vi "LVClass_CameraSet GetGenericParameterBoolValue.vi"(0 "CameraSet.lvclass":refnum<class "CameraSet.lvclass">, 5 "parameter_name":string, 7 "DefaultFactorySet":bool, 11 "error in (no error)":errorcluster) -> (4 "CameraSet.lvclass":refnum<class "CameraSet.lvclass">, 6 "Value":bool, 15 "error out":errorcluster)   [LabVIEW 2020, in "CameraSet.lvclass"]
doc: "Camera parameter value getter for parameter of type boolean.\n\n<B>camera_setIn</B> : CameraSet object.\n<B>camera_setOut</B> : CameraSet object.\n<B>parameter_name</B> : Parameter name.\n<B>value</B> : Parameter value."
uses:
  CameraSet.lvclass
  CameraSet.lvclass/CameraSet.ctl
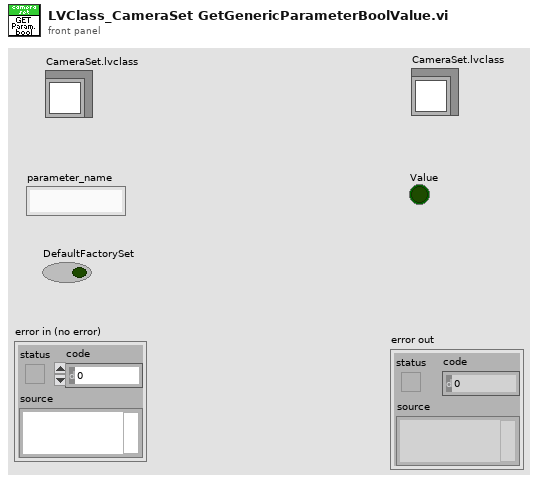
[diagram p1: front panel]
types:
  T1 = typedef "ClassID.ctl" = i64
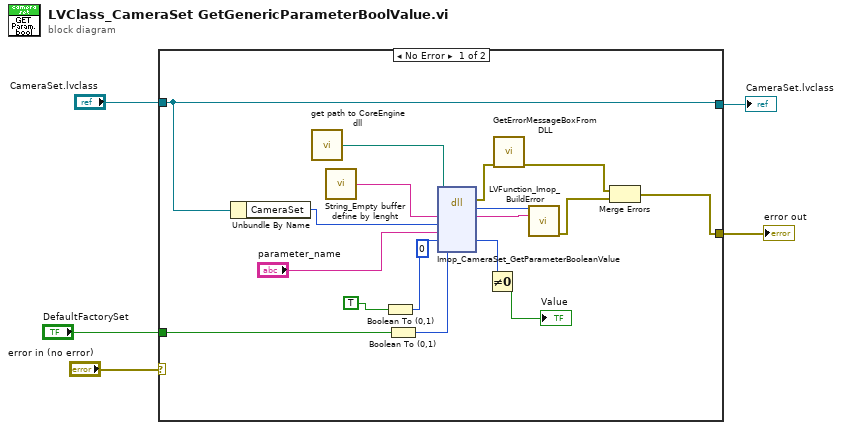
[diagram p0: block diagram]
diagram:
  n1 = case shown="No Error" "error in (no error)" {
    selector: "error in (no error)" -> [_ w23]
    tunnel: "CameraSet.lvclass" -> [w12 w24]
    tunnel: [w12 w24] -> w3
    tunnel: [w10 w23] -> w2
    tunnel: "DefaultFactorySet" -> [w6 _]
    frame No Error {
      (unwired) u8 0 ("DefaultFactorySet")
      n2 = Unbundle By Name(w12) -> ("CameraSet"=w11:T1)
      n3 = call "get path to CoreEngine dll.vi"() -> ("path to c_interface_vc100.dll"=w18:path)  [unwired: 12 in, 3 out]
      n4 = call "String_Empty buffer define by lenght.vi"() -> ("Empty buffer"=w20:string)  [unwired: 1 in]
      n5 = Boolean To (0,1)(Boolean=TRUE) -> (0, 1=w15:i16)
      n6 = Boolean To (0,1)(Boolean=w6) -> (0, 1=w7:i16)
      n7 = dll-call lib="D:/soft/HASO_v3/SVN_trunk/ImOpCoreEngine4_LV2011/DLLs/c_interface_vc100.dll" fn="Imop_CameraSet_GetParameterBooleanValue"(path in=w18, "message"=w20, "objet"=w11, "parameter_name"="parameter_name", "value"=w15, "DefaultFactorySet"=w7) -> (error out=w17:errorcluster, "return type"=w22:i32, "message"=w21:string, "value"=w14:u8)  [unwired: 5 in, 1 out]
      n8 = Not Equal To 0?(x=w14) -> (x != 0?=→"Value":bool)
      n9 = call "GetErrorMessageBoxFromDLL.vi"("error IN"=w17) -> ("error OUT"=w9:errorcluster)  [unwired: 10 in]
      n10 = call "LVFunction_Imop_BuildError.vi"("code"=w22, "String to Prepend to source (\"\")"=w21) -> ("error out"=w8:errorcluster)  [unwired: 13 in]
      n11 = Merge Errors(w9, w8) -> (w10:errorcluster)
    }
    frame Error {
    }
  }
  "CameraSet.lvclass" <- w3
  "error out" <- w2
